vi "EdgeProcessing.vi"() -> ()   [LabVIEW 2019]
uses:
  <vilib>/userDefined/High Color/IMAQdx.ctl
  <vilib>/vision/driver/NI_Vision_Acquisition_Software.lvlib
  <vilib>/vision/NI_Vision_Development_Module.lvlib
panel:
  in  "Filter Parameters":T1={"Sigma"=1.0, "HThresh"=0.7, "LThres"=0.2, "WindowSize"=9} {"LThres" min=0 max=1 format="%.2f"; "HThresh" min=0 max=1 format="%.2f"; "Sigma" min=0 max=1 format="%.2f"}
  out "Image 4":T2(plugin-control)
  out "Image":T2(plugin-control)
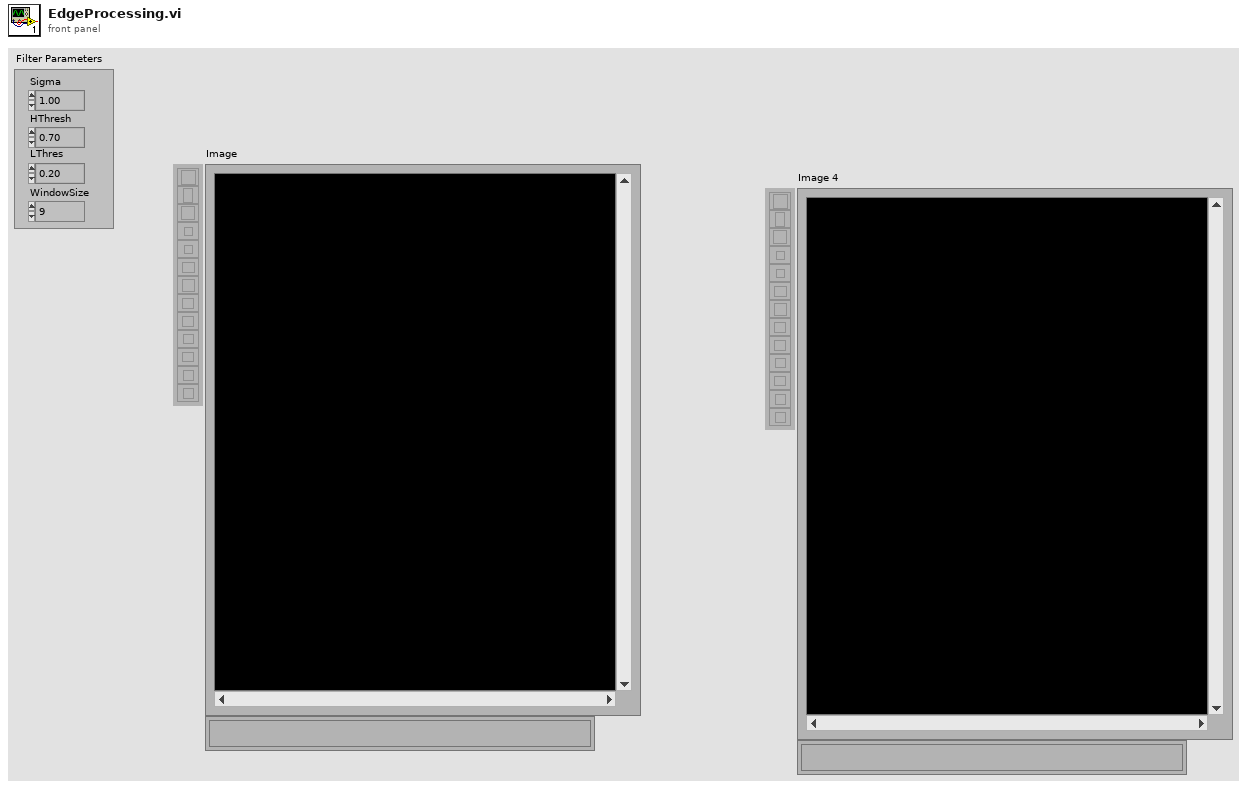
[diagram p1: front panel]
types:
  T1 = cluster{"Sigma":sgl, "HThresh":sgl, "LThres":sgl, "WindowSize":i32}
  T2 = typedef "IMAQ Image.ctl" = refnum<image>
  T3 = typedef "IMAQdx.ctl" = refnum<k21>
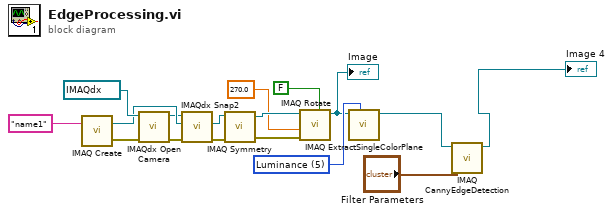
[diagram p0: block diagram]
diagram:
  w5 = 5 items=["Red", "Green", "Blue", "Hue", "Saturation", "Luminance", "Value", "Intensity"] ("Color Plane")
  n1 = call "IMAQ Create"("Image Name"="name1") -> ("New Image"=w15:T2, "error out"=w13:errorcluster)  [unwired: 4 in]
  n2 = call <vilib>:"IMAQdx Open Camera.vi"("error in"=w13, "Session In"=T3 "cam0") -> ("error out"=w16:errorcluster, "Session Out"=w14:T3)  [unwired: 8 in]
  n3 = call <vilib>:"IMAQdx Snap2.vi"("error in"=w16, "Image In"=w15, "Session In"=w14) -> ("error out"=w8:errorcluster, "Image Out"=w9:T2)  [unwired: 6 in, 1 out]
  n4 = call "IMAQ Symmetry"("error in (no error)"=w8, "Image Src"=w9) -> ("error out"=w7:errorcluster, "Image Dst Out"=w12:T2)  [unwired: 3 in]
  n5 = call "IMAQ Rotate"("Maintain Size"=FALSE, "error in (no error)"=w7, "Angle (degrees)"=sgl 270.0, "Image Src"=w12) -> ("Image Dst Out"=w4:T2)  [unwired: 6 in, 1 out]
  "Image" <- w4
  n6 = call "IMAQ ExtractSingleColorPlane"("Color Plane"=w5, "Image Src"=w4) -> ("Image Dst Out"=w3:T2)  [unwired: 8 in, 1 out]
  n7 = call "IMAQ CannyEdgeDetection"("Image Src"=w3, "Filter Parameters"="Filter Parameters") -> ("Image Dst Out"=→"Image 4":T2)  [unwired: 6 in, 1 out]
